vi "Acoustic Noise - Debug.vi"(0 "TSM context":T4, 1 "Capture Duration (s)":dbl, 5 "Minimum Frequency (Hz)":dbl=20.0 format="%#_13g", 7 "Maximum Frequency(Hz)":dbl=200.0 format="%#_13g", 9 "Window(Rectangle)":T3 items=["Rectangle"=0, "Hanning"=1, "Hamming"=2, "Blackman-Harris"=3, "Exact Blackman"=4, "Blackman"=5, "Flat Top"=6, "4 Term B-Harris "=7, "7 Term B-Harris"=8, "Low Sidelobe"=9, "Blackman Nuttall"=11, "Triangle"=30, "Bartlett-Hanning"=31, "Bohman"=32, "Parzen"=33, "Welch"=34, "Kaiser"=60, "Dolph-Chebyshev"=61, "Gaussian"=62]) -> (15 "error out":errorcluster)   [LabVIEW 2020]
doc: "Acoustic Noise VI help to capture the noise waveform from the reference mic and the DUT, and calculate the A-weighted noise (dBA) for those waveforms"
uses:
  <vilib>/NI_TestStand_SemiconductorModule/NI_TestStand_Semiconductor_Module.lvlibp/PinMap/General/SemiconductorModuleContext.ctl
  <vilib>/Analysis/4window.llb/windowTd.ctl
  <vilib>/measure/maspectr.llb/FFT Power Spectrum and PSD for N Chan.vi
  <vilib>/Analysis/1siggen.llb/Ramp Pattern by Delta.vi
  <vilib>/measure/NI_MAPro.lvlib
  <vilib>/Analysis/NI_AALPro.lvlib
  <vilib>/Analysis/NI_AALBase.lvlib
  <vilib>/NI_TestStand_SemiconductorModule/NI_TestStand_Semiconductor_Module.lvlibp
panel:
  in  "dB Pa(T) / dB V(F)":bool
  in  "restart averaging (F)":bool
  in  "averaging parameters":T1={"averaging mode"=enum."RMS averaging", "weighting mode"=enum."Exponential", "number of averages"=5}
  out "XY Graph":T2(graph)
  in  "stop":bool
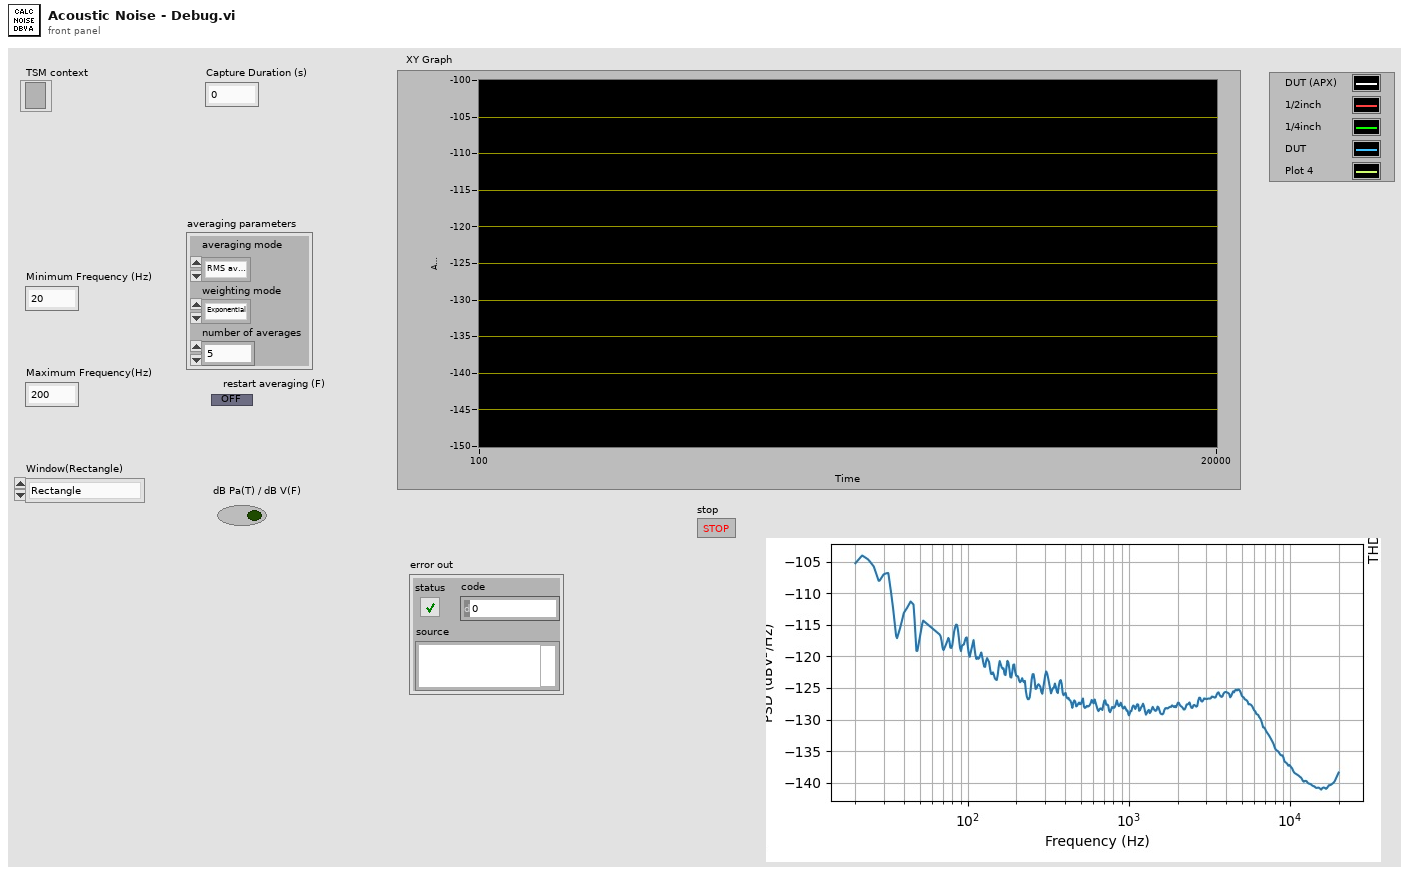
[diagram p1: front panel]
types:
  T1 = cluster{"averaging mode":enum16{"No averaging", "Vector averaging", "RMS averaging", "Peak hold"}, "weighting mode":enum16{"Linear", "Exponential"}, "number of averages":u32}
  T2 = cluster{"Ramp Pattern":dbl[], "magnitude":dbl[]}[]
  T3 = typedef "NI_AALPro.lvlib/windowTd.ctl" = u32
  T4 = typedef "NI_TestStand_Semiconductor_Module.lvlibp/SemiconductorModuleContext.ctl" = refnum<k7>
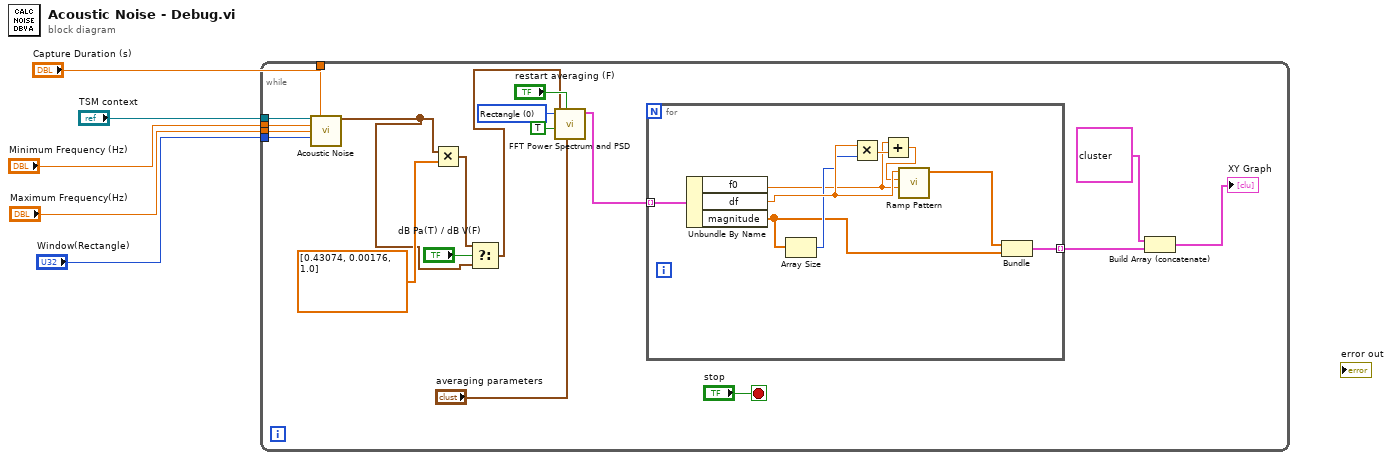
[diagram p0: block diagram]
diagram:
  n1 = while {
    tunnel: "TSM context" -> [w24]
    tunnel: "Capture Duration (s)" -> [w23]
    tunnel: "Minimum Frequency (Hz)" -> [w22]
    tunnel: "Maximum Frequency(Hz)" -> [w21]
    tunnel: "Window(Rectangle)" -> [w20]
    stop <- "stop" stop-if-true
    w18 = T3 0 items=["Rectangle"=0, "Hanning"=1, "Hamming"=2, "Blackman-Harris"=3, "Exact Blackman"=4, "Blackman"=5, "Flat Top"=6, "4 Term B-Harris "=7, "7 Term B-Harris"=8, "Low Sidelobe"=9, "Blackman Nuttall"=11, "Triangle"=30, "Bartlett-Hanning"=31, "Bohman"=32, "Parzen"=33, "Welch"=34, "Kaiser"=60, "Dolph-Chebyshev"=61, "Gaussian"=62] ("window")
    n2 = call "Acoustic Noise.vi"("TSM context"=w24, "Capture Duration (s)"=w23, "Minimum Frequency (Hz)"=w22, "Maximum Frequency(Hz)"=w21, "Window(Rectangle)"=w20) -> ("Per-Site Waveform Out"=w7:waveform(dbl)[])  [unwired: 9 in, 1 out]
    n3 = Multiply(x=w7, y=dbl[] [0.43074, 0.00176, 1.0]) -> (x*y=w8:waveform(dbl)[])
    n4 = Select(t=w8, s="dB Pa(T) / dB V(F)", f=w7) -> (s? t:f=w6:waveform(dbl)[])
    n5 = call-poly <vilib>:"FFT Power Spectrum and PSD.vi"("averaging parameters"="averaging parameters", "restart averaging (F)"="restart averaging (F)", "dB On (F)"=TRUE, "window"=w18, "time signals"=w6) -> ("Power Spectrum / PSD"=w15:cluster{"f0":dbl, "df":dbl, "magnitude":dbl[]}[])  [unwired: 3 in, 3 out]
    n6 = for {
      tunnel: w15 -> [w33] mode=indexing
      tunnel: [w25] -> w14 mode=indexing
      n7 = Unbundle By Name(w33) -> ("f0"=w29:dbl, "df"=w32:dbl, "magnitude"=w26:dbl[])
      n8 = Array Size(array=w26) -> (size(s)=w31:i32)
      n9 = Multiply(x=w32, y=w31) -> (x*y=w30:dbl)
      n10 = Add(x=w29, y=w30) -> (x+y=w28:dbl)
      n11 = call-poly <vilib>:"Ramp Pattern.vi"("start"=w29, "end"=w28, "delta"=w32) -> ("Ramp Pattern"=w27:dbl[])  [unwired: 6 in, 2 out]
      n12 = Bundle("Ramp Pattern"=w27, "magnitude"=w26) -> (w25:cluster{"Ramp Pattern":dbl[], "magnitude":dbl[]})  [unwired: 1 in]
    }
    n13 = Build Array (concatenate)(cluster{dbl[], dbl[]} {array[500 elements], array[500 elements]} ("XY Graph"), w14) -> (→"XY Graph":T2)
  }
